vi "Write Process Action Name.vi"(8 "error in (no error)":errorcluster, 10 "Process Action Name":string[](array[string]), 11 "MPC_Laser Marked in":refnum<class "MPC_Laser Marked.lvclass">) -> (0 "error out":errorcluster, 3 "MPC_Laser Marked out":refnum<class "MPC_Laser Marked.lvclass">)   [LabVIEW 2019, in "MPC_Laser Marked.lvclass"]
uses:
  MPC_Laser Marked.lvclass
  MPC_Laser Marked.lvclass/MPC_Laser Marked.ctl
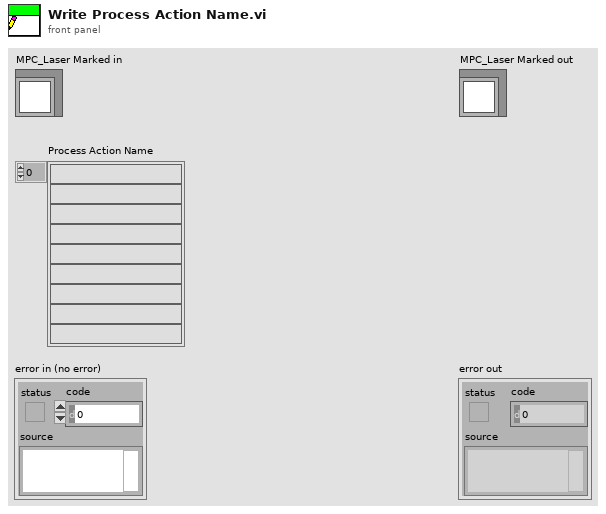
[diagram p1: front panel]
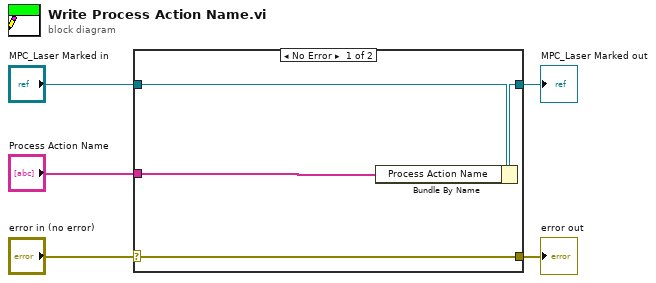
[diagram p0: block diagram]
diagram:
  n1 = case shown="No Error" "error in (no error)" {
    selector: "error in (no error)" -> [w9 w10]
    tunnel: [w9 w10] -> w4
    tunnel: [w7 w11] -> w2
    tunnel: "MPC_Laser Marked in" -> [w8 w11]
    tunnel: "Process Action Name" -> [w6 _]
    frame No Error {
      n2 = Bundle By Name(cluster=w8, "Process Action Name"=w6) -> (w7:refnum<class "MPC_Laser Marked.lvclass">)
    }
    frame Error {
    }
  }
  "error out" <- w4
  "MPC_Laser Marked out" <- w2
